vi "Reachable Time Finished.vi"(1 "Angle Displacement":dbl, 2 "Max Acceleration":dbl, 3 "Reachable Angular Velocity":dbl) -> (0 "Reachable Time Finished":dbl)   [LabVIEW 2015]
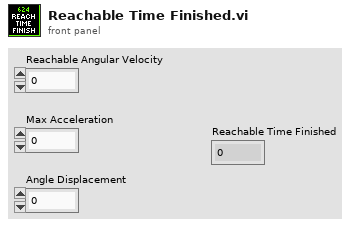
[diagram p1: front panel]
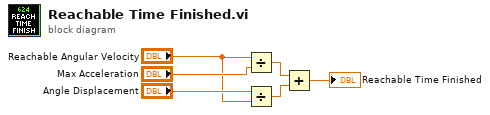
[diagram p0: block diagram]
diagram:
  n1 = Divide(x="Reachable Angular Velocity", y="Max Acceleration") -> (x/y=w2:dbl)
  n2 = Divide(x="Angle Displacement", y="Reachable Angular Velocity") -> (x/y=w3:dbl)
  n3 = Add(x=w2, y=w3) -> (x+y=→"Reachable Time Finished":dbl)
